vi "IniWrite.vi"(7 "section":string caption="段", 8 "error in (no error)":errorcluster caption="错误输入（无错误）", 10 "控件引用":refnum<vi>, 11 "Ini.In":T1 caption="引用句柄") -> (0 "error out":errorcluster caption="错误输出", 3 "Ini.Out":T1 caption="refnum out")   [LabVIEW 2012, in "IniReader&WriterForControl.lvlib"]
uses:
  IniReader&WriterForControl.lvlib
  <vilib>/Utility/config.llb/Config Data RefNum.ctl
  <vilib>/Utility/config.llb/Write Key (String).vi
  <vilib>/Utility/config.llb/Write Key (Double).vi
  <vilib>/Utility/config.llb/Write Key (Path).vi
  <vilib>/Utility/config.llb/Write Key (Boolean).vi
  <vilib>/Utility/config.llb/NI_LVConfig.lvlib
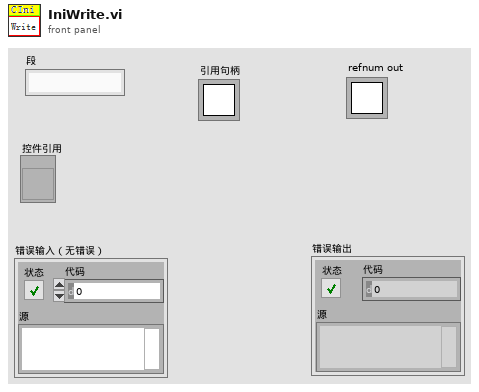
[diagram p1: front panel]
types:
  T1 = typedef "NI_LVConfig.lvlib/Config Data RefNum.ctl" = refnum<k1>
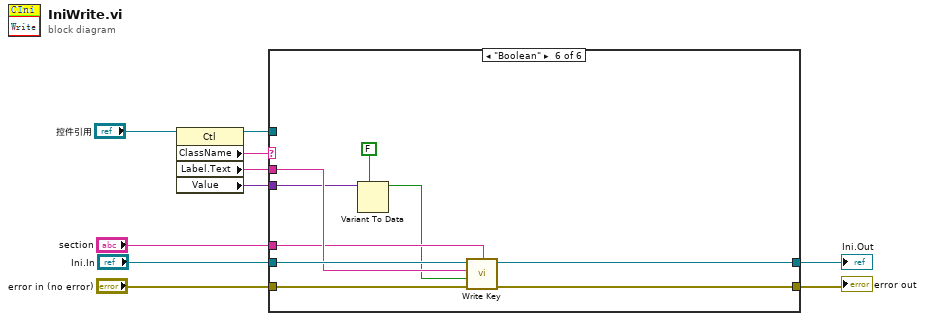
[diagram p0: block diagram]
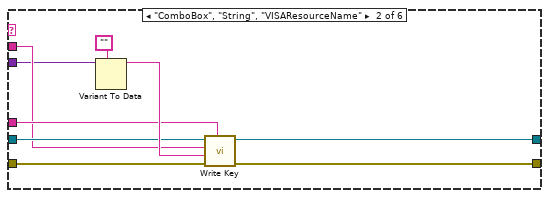
[diagram p3: hidden frame]
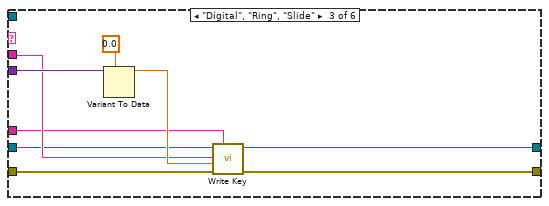
[diagram p4: hidden frame]
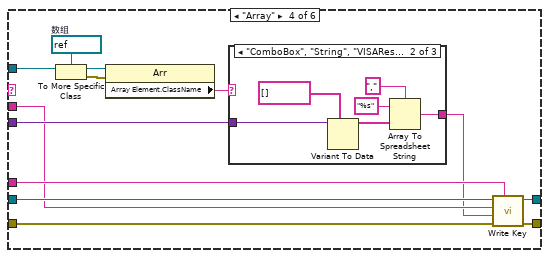
[diagram p5: hidden frame]
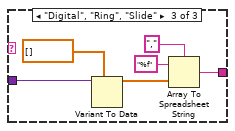
[diagram p7: hidden frame]
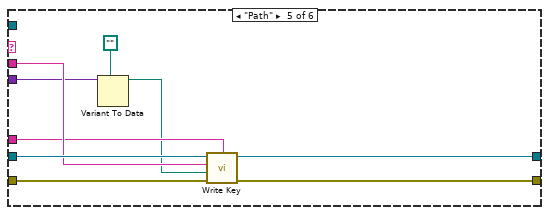
[diagram p8: hidden frame]
diagram:
  n1 = property class="Ctl"(reference="控件引用") -> (reference out=w9:refnum<vi>, "ClassName"=w10:string, "Label.Text"=w7:string, "Value"=w2:variant)  [unwired: 1 in, 1 out]
  n2 = case shown="\"Boolean\"" w10 {
    tunnel: w9 -> [_ _ _ w38 _ _]
    tunnel: "Ini.In" -> [w12 w16 w25 w41 w64 w73]
    tunnel: w7 -> [_ w15 w27 w32 w63 w72]
    tunnel: "error in (no error)" -> [w11 w20 w29 w43 w62 w71]
    tunnel: [w11 w19 w24 w40 w61 w70] -> w3
    tunnel: [w12 w18 w23 w39 w60 w69] -> w4
    tunnel: w2 -> [_ w14 w28 w33 w58 w67]
    tunnel: "section" -> [_ w17 w26 w42 w59 w68]
    frame "假", Default {
    }
    frame "ComboBox", "String", "VISAResourceName" {
      n3 = Variant To Data(type="", Variant=w14) -> (data=w21:string)  [unwired: 1 in, 1 out]
      n4 = call-poly <vilib>:"Write Key.vi"("section"=w17, "error in (no error)"=w20, "value"=w21, "key"=w15, "refnum"=w16) -> ("error out"=w19:errorcluster, "refnum out"=w18:T1)  [unwired: 4 in, 1 out]
    }
    frame "Digital", "Ring", "Slide" {
      n5 = Variant To Data(type=0.0, Variant=w28) -> (data=w30:dbl)  [unwired: 1 in, 1 out]
      n6 = call-poly <vilib>:"Write Key.vi"("section"=w26, "error in (no error)"=w29, "value"=w30, "key"=w27, "refnum"=w25) -> ("error out"=w24:errorcluster, "refnum out"=w23:T1)  [unwired: 4 in, 1 out]
    }
    frame "Array" {
      w37 = refnum<vi> refnum  # 数组
      n7 = To More Specific Class(target class=w37, reference=w38) -> (specific class reference=w36:refnum<vi>, error out=w35:errorcluster)  [unwired: 1 in]
      n8 = property class="Arr"(reference=w36, error in=w35) -> ("Array Element.ClassName"=w34:string)  [unwired: 2 out]
      n9 = case shown="\"ComboBox\", \"String\", \"VISAResourceName\"" w34 {
        tunnel: w33 -> [_ w49 w55]
        tunnel: [_ w44 w50] -> w31
        frame "假", Default {
        }
        frame "ComboBox", "String", "VISAResourceName" {
          n10 = Variant To Data(type=string[] [], Variant=w49) -> (data=w47:string[])  [unwired: 1 in, 1 out]
          n11 = Array To Spreadsheet String(delimiter (Tab)="," ("分隔符(Tab)"), array=w47, 3:"%s" ("格式字符串")) -> (spreadsheet string=w44:string)
        }
        frame "Digital", "Ring", "Slide" {
          n12 = Variant To Data(type=dbl[] [], Variant=w55) -> (data=w51:dbl[])  [unwired: 1 in, 1 out]
          n13 = Array To Spreadsheet String(delimiter (Tab)="," ("分隔符(Tab)"), array=w51, 3:"%f" ("格式字符串")) -> (spreadsheet string=w50:string)
        }
      }
      n14 = call-poly <vilib>:"Write Key.vi"("section"=w42, "error in (no error)"=w43, "value"=w31, "key"=w32, "refnum"=w41) -> ("error out"=w40:errorcluster, "refnum out"=w39:T1)  [unwired: 4 in, 1 out]
    }
    frame "Path" {
      n15 = Variant To Data(type=path "", Variant=w58) -> (data=w56:path)  [unwired: 1 in, 1 out]
      n16 = call-poly <vilib>:"Write Key.vi"("section"=w59, "error in (no error)"=w62, "value"=w56, "key"=w63, "refnum"=w64) -> ("error out"=w61:errorcluster, "refnum out"=w60:T1)  [unwired: 4 in, 1 out]
    }
    frame "Boolean" {
      n17 = Variant To Data(type=FALSE, Variant=w67) -> (data=w65:bool)  [unwired: 1 in, 1 out]
      n18 = call-poly <vilib>:"Write Key.vi"("section"=w68, "error in (no error)"=w71, "value"=w65, "key"=w72, "refnum"=w73) -> ("error out"=w70:errorcluster, "refnum out"=w69:T1)  [unwired: 4 in, 1 out]
    }
  }
  "error out" <- w3
  "Ini.Out" <- w4
